vi "Error_AddCallChain.vi"(5 "error in (no error)":errorcluster) -> (19 "error out":errorcluster)   [LabVIEW 2020]
doc: "If error in, this VI adds the source of the calling VI of this VI."
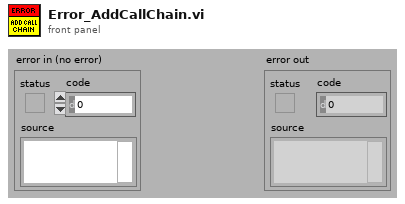
[diagram p1: front panel]
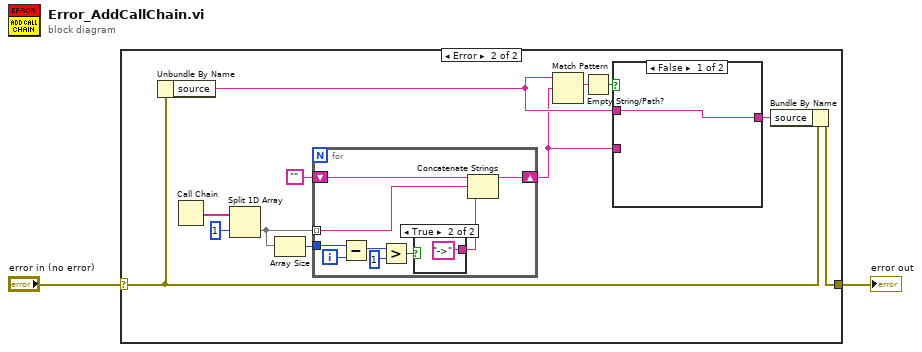
[diagram p0: block diagram]
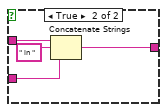
[diagram p3: hidden frame]
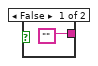
[diagram p4: hidden frame]
diagram:
  n1 = case shown="Error" "error in (no error)" {
    selector: "error in (no error)" -> [w3 w4]
    tunnel: [w3 w15] -> w2
    frame No Error {
    }
    frame Error {
      n2 = Unbundle By Name(w4) -> ("source"=w7:string)
      n3 = Call Chain() -> (call chain=w14:string[])
      n4 = Split 1D Array(array=w14, index=1) -> (second subarray=w12:string[])  [unwired: 1 out]
      n5 = Array Size(array=w12) -> (size(s)=w11:i32)
      n6 = for {
        shift-right: [w21] -> w6
        shift-left: "" -> [w24]
        tunnel: w12 -> [w22] mode=indexing
        tunnel: w11 -> [w29]
        i -> [w28]
        n7 = Subtract(x=w29, y=w28) -> (x-y=w27:i32)
        n8 = Greater?(x=w27, y=1) -> (0:w25:bool)
        n9 = case shown="True" w25 {
          tunnel: ["" "->"] -> w23
          frame False {
          }
          frame True {
          }
        }
        n10 = Concatenate Strings(w24, w22, w23) -> (w21:string)
      }
      n11 = Match Pattern(string=w7, regular expression=w6) -> (match substring=w9:string)  [unwired: 4 out]
      n12 = Empty String/Path?(string/path=w9) -> (empty?=w8:bool)
      n13 = case shown="False" w8 {
        tunnel: w7 -> [w16 w19]
        tunnel: w6 -> [_ w18]
        tunnel: [w16 w17] -> w5
        frame False {
        }
        frame True {
          n14 = Concatenate Strings(w19, " in " ("Substring"), w18) -> (w17:string)
        }
      }
      n15 = Bundle By Name(cluster=w4, "source"=w5) -> (w15:errorcluster)
    }
  }
  "error out" <- w2
